vi "set_or_clear_reference_object.vi"(1 "input cluster":T3) -> (0 "last acquired buffer out":i32)   [LabVIEW 2015]
uses:
  <vilib>/vision/Avi1.llb/AviRefnum.ctl
  <vilib>/userdefined/High Color/IMAQdx.ctl
  MWT.dll
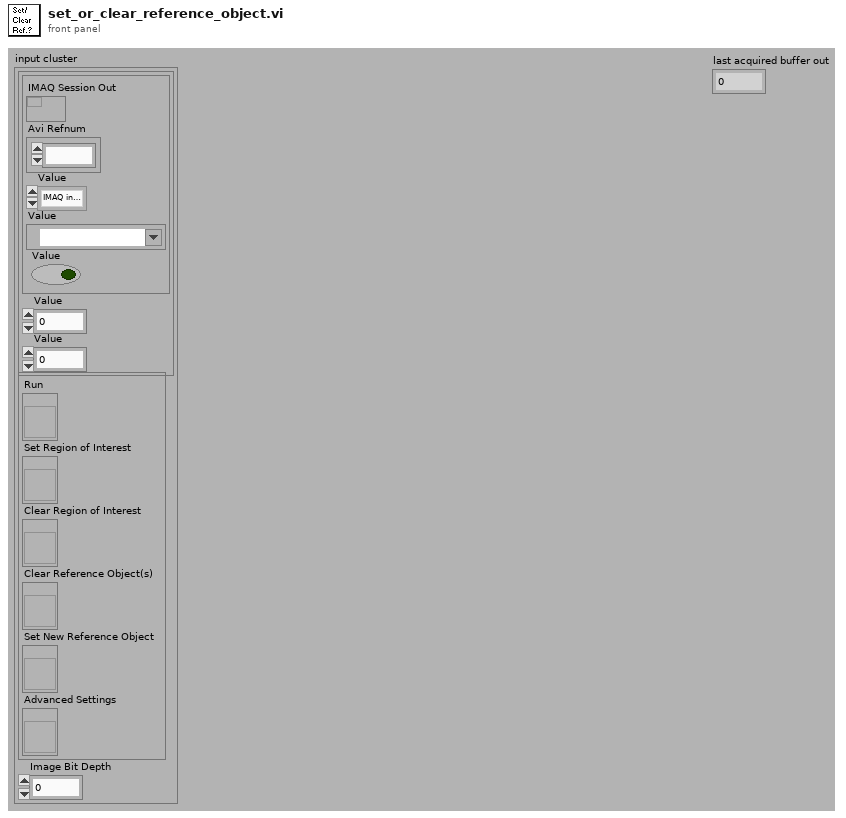
[diagram p1: front panel]
types:
  T1 = typedef "AviRefnum.ctl" = refnum<k1>
  T2 = typedef "IMAQdx.ctl" = refnum<k21>
  T3 = cluster{cluster{cluster{"IMAQ Session Out":refnum<k11>, "Avi Refnum":T1, "Value":enum32{"IMAQ interface", "IMAQdx interface", "AVI file"}, "Value":T2, "Value":bool}, "Value":i32, "Value":i32}, cluster{"Run":refnum<vi>, "Set Region of Interest":refnum<vi>, "Clear Region of Interest":refnum<vi>, "Clear Reference Object(s)":refnum<vi>, "Set New Reference Object":refnum<vi>, "Advanced Settings":refnum<vi>}, "Image Bit Depth":u32}
  T4 = cluster{cluster{"IMAQ Session Out":refnum<k11>, "Avi Refnum":T1, "Value":enum32{"IMAQ interface", "IMAQdx interface", "AVI file"}, "Value":T2, "Value":bool}, "Value":i32, "Value":i32}
  T5 = cluster{"Run":refnum<vi>, "Set Region of Interest":refnum<vi>, "Clear Region of Interest":refnum<vi>, "Clear Reference Object(s)":refnum<vi>, "Set New Reference Object":refnum<vi>, "Advanced Settings":refnum<vi>}
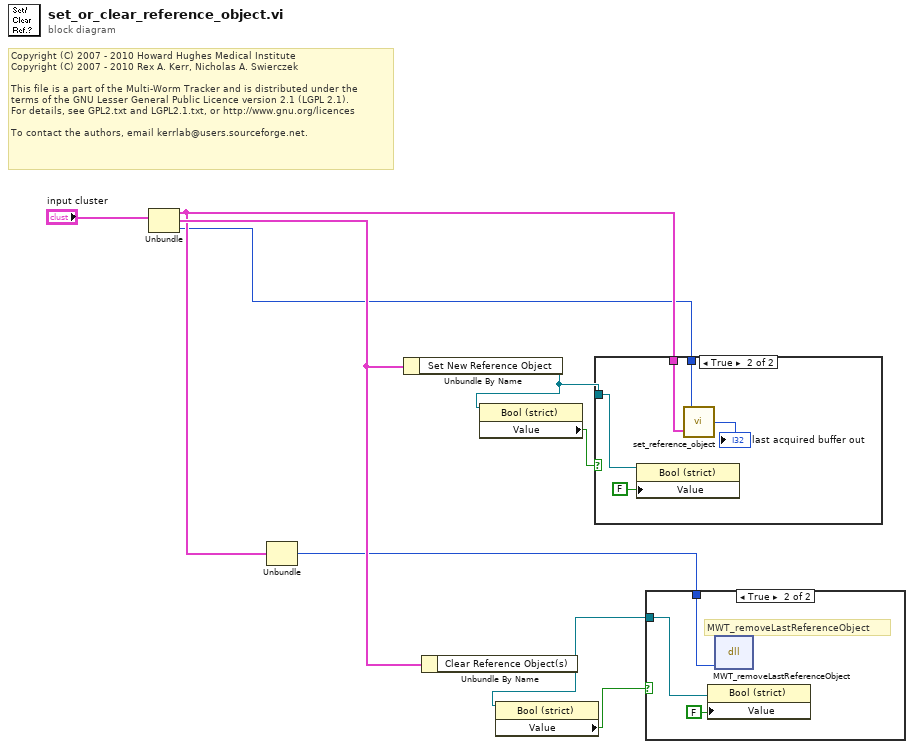
[diagram p0: block diagram]
diagram:
  # "Copyright (C) 2007 - 2010 Howard Hughes Medical Institute\nCopyright (C) 2007 - 2010 Rex A. Kerr, Nicholas A. Swierczek\n \nThis file is a part of the Multi-Worm Tracker and is distributed under the\nterms of the GNU Lesser General Public Licence version 2.1 (LGPL 2.1).\nFor details, see GPL2.txt and LGPL2.1.txt, or http://www.gnu.org/licences\n \nTo contact the authors, email kerrlab@users.sourceforge.net."
  n1 = Unbundle("input cluster") -> (w3:T4, w5:T5, "Image Bit Depth"=w2:u32)
  n2 = Unbundle(w3) -> ("Value"=w4:i32)  [unwired: 2 out]
  n3 = Unbundle By Name(w5) -> ("Set New Reference Object"=w8:refnum<vi>)
  n4 = Unbundle By Name(w5) -> ("Clear Reference Object(s)"=w7:refnum<vi>)
  n5 = property class="Bool (strict)"(reference=w8) -> ("Value"=w9:bool)  [unwired: 1 in, 2 out]
  n6 = property class="Bool (strict)"(reference=w7) -> ("Value"=w6:bool)  [unwired: 1 in, 2 out]
  n7 = case shown="True" w9 {
    tunnel: w8 -> [_ w14]
    tunnel: w3 -> [_ w12]
    tunnel: w2 -> [_ w10]
    frame False {
    }
    frame True {
      n8 = property class="Bool (strict)"(reference=w14, "Value"=FALSE ("OK Button")) -> ()  [unwired: 1 in, 2 out]
      n9 = call "set_reference_object.vi"("camera cluster"=w12, "bit depth"=w10) -> ("last acquired buffer out"=→"last acquired buffer out":i32)
    }
  }
  n10 = case shown="True" w6 {
    tunnel: w7 -> [_ w16]
    tunnel: w4 -> [_ w17]
    frame False {
    }
    frame True {
      # "MWT_removeLastReferenceObject"
      n11 = property class="Bool (strict)"(reference=w16, "Value"=FALSE ("OK Button")) -> ()  [unwired: 1 in, 2 out]
      n12 = dll-call lib="C:/Users/ramasamyl/Desktop/MWT/MWT.dll" fn="MWT_removeLastReferenceObject"("handle"=w17) -> ()  [unwired: 5 in, 2 out]
    }
  }
